vi "searchLibItem.vi"(8 "error in (no error)":errorcluster, 9 "regExpr":string, 10 "Owned Items[]":refnum<vi>[](array[refnum]), 11 "LibReader in":refnum<class "LibReader.lvclass">) -> (0 "error out":errorcluster, 1 "ProjectItem Refnum":refnum<vi>, 2 "found":bool, 3 "LibReader out":refnum<class "LibReader.lvclass">)   [LabVIEW 2018, in "LibReader.lvclass"]
doc: "Search the item in lvlib."
uses:
  LibReader.lvclass
  <vilib>/regexp/Match Regular Expression.xnode
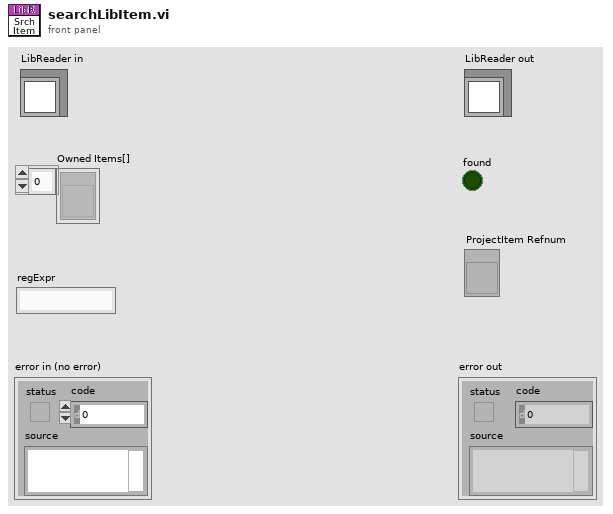
[diagram p1: front panel]
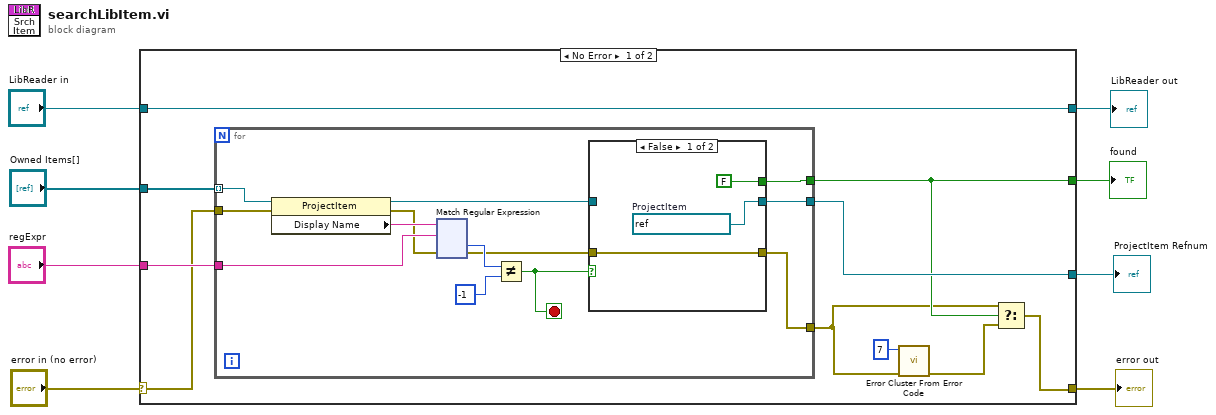
[diagram p0: block diagram]
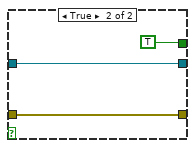
[diagram p2: hidden frame]
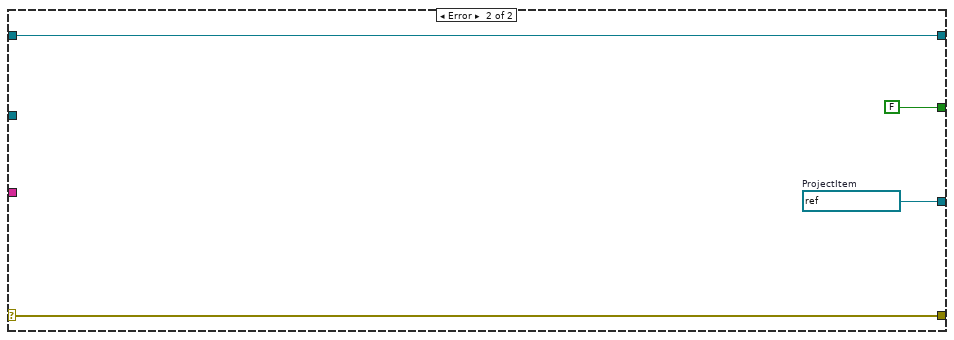
[diagram p3: hidden frame]
diagram:
  n1 = case shown="No Error" "error in (no error)" {
    selector: "error in (no error)" -> [w16 w155]
    tunnel: [w12 w155] -> w7
    tunnel: [w18 w154] -> w4
    tunnel: "LibReader in" -> [w18 w154]
    tunnel: "regExpr" -> [w17 _]
    tunnel: [w13 FALSE] -> w5
    tunnel: "Owned Items[]" -> [w15 _]
    tunnel: [w14 w152] -> w1
    frame No Error {
      n2 = for {
        tunnel: w15 -> [w31] mode=indexing
        tunnel: w16 -> [w29]
        tunnel: w17 -> [w28]
        tunnel: [w21] -> w13
        tunnel: [w20] -> w9
        tunnel: [w19] -> w14
        stop <- w24 stop-if-true
        n3 = property class="ProjectItem"(reference=w31, error in=w29) -> (reference out=w23:refnum<vi>, error out=w25:errorcluster, "Display Name"=w30:string)
        n4 = xnode "Match Regular Expression"("input string"=w30, "regular expression"=w28, "error in"=w25) -> ("offset past match"=w27:i32, "error out"=w22:errorcluster)  [unwired: 3 in, 3 out]
        n5 = Not Equal?(x=w27, y=-1) -> (x != y?=w24:bool)
        n6 = case shown="False" w24 {
          tunnel: w23 -> [_ w35]
          tunnel: w22 -> [w34 w36]
          tunnel: [w34 w36] -> w20
          tunnel: [FALSE TRUE] -> w21
          tunnel: [w32 w35] -> w19
          frame False {
            w32 = refnum<vi> refnum  # ProjectItem
          }
          frame True {
          }
        }
      }
      n7 = call <vilib>:"Error Cluster From Error Code.vi"("error in (no error)"=w9, "error code (0)"=7) -> ("error out"=w11:errorcluster)  [unwired: 7 in]
      n8 = Select(t=w9, s=w13, f=w11) -> (s? t:f=w12:errorcluster)
    }
    frame Error {
      w152 = refnum<vi> refnum  # ProjectItem
    }
  }
  "error out" <- w7
  "LibReader out" <- w4
  "found" <- w5
  "ProjectItem Refnum" <- w1
